vi "(Sub) Run Butten Enable.vi"(0 "Test Group":bool[](array[boolean]), 1 "G1.Comm":bool caption="G1. Comm", 2 "G1.System":bool caption="G1. System", 3 "G2.Comm":bool caption="G2. Comm", 4 "G2.System":bool caption="G2. System", 5 "G3.Comm":bool caption="G3. Comm", 6 "G3.System":bool caption="G3. System", 7 "error in (no error)":errorcluster caption="에러 입력(에러 없음)") -> (21 "E/Dnable":T1(ring), 27 "error out":errorcluster caption="에러 출력")   [LabVIEW 2017]
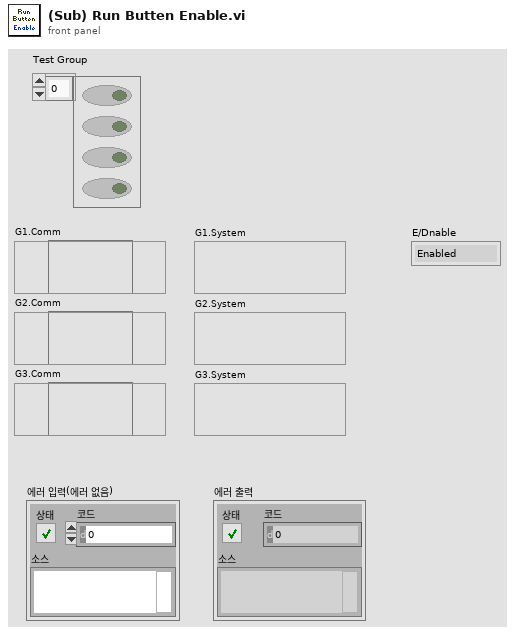
[diagram p1: front panel]
types:
  T1 = enum8{"Enabled", "Disabled", "Disabled and Grayed Out"}
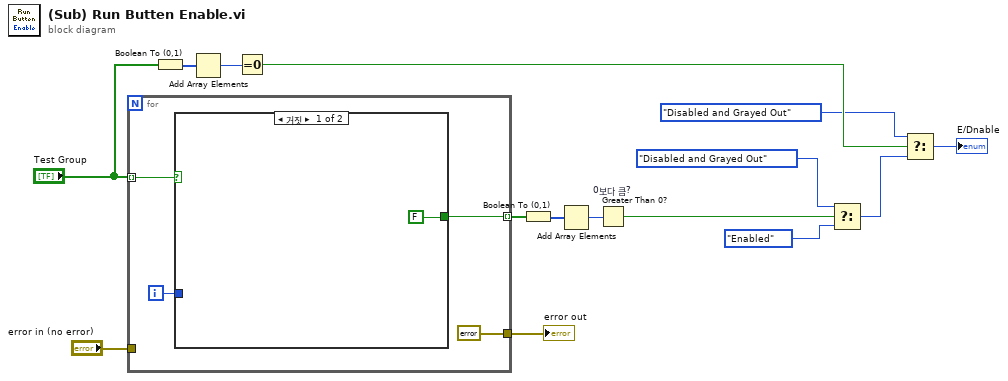
[diagram p0: block diagram]
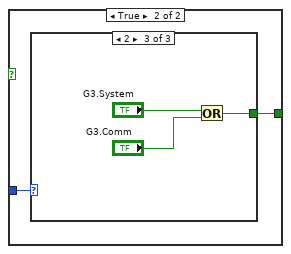
[diagram p2: hidden frame]
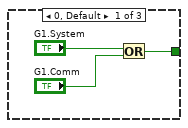
[diagram p3: hidden frame]
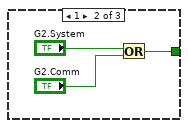
[diagram p4: hidden frame]
diagram:
  n1 = for {
    tunnel: "Test Group" -> [w19] mode=indexing
    tunnel: [w17] -> w15 mode=indexing
    tunnel: "error in (no error)" -> [_]
    tunnel: [errorcluster {"status"=FALSE, "code"=0, "source"=""} ("에러 상수")] -> w12
    i -> [w18]
    n2 = case shown="거짓" w19 {
      tunnel: w18 -> [_ w22]
      tunnel: [FALSE w21] -> w17
      frame False {
      }
      frame True {
        n3 = case shown="2" w22 {
          tunnel: [w25 w28 w31] -> w21
          frame 0, Default {
            n4 = Or(x="G1.System", y="G1.Comm") -> (x .or. y?=w25:bool)
          }
          frame 1 {
            n5 = Or(x="G2.System", y="G2.Comm") -> (x .or. y?=w28:bool)
          }
          frame 2 {
            n6 = Or(x="G3.System", y="G3.Comm") -> (x .or. y?=w31:bool)
          }
        }
      }
    }
  }
  "error out" <- w12
  n7 = Boolean To (0,1)(Boolean="Test Group") -> (0, 1=w7:i16[])
  n8 = Add Array Elements(numeric array=w7) -> (sum=w5:i16)
  n9 = Equal To 0?(x=w5) -> (x = 0?=w3:bool)
  n10 = Boolean To (0,1)(Boolean=w15) -> (0, 1=w8:i16[])
  n11 = Add Array Elements(numeric array=w8) -> (sum=w14:i16)
  n12 = Greater Than 0? "0보다 큼?"(x=w14) -> (x > 0?=w9:bool)
  n13 = Select(t=T1."Disabled and Grayed Out" ("비활성화"), s=w9, f=T1."Enabled" ("비활성화")) -> (s? t:f=w4:T1)
  n14 = Select(t=T1."Disabled and Grayed Out" ("비활성화"), s=w3, f=w4) -> (s? t:f=→"E/Dnable":T1)
